vi "Configure PID Differential Time.vi"(8 "error in (no error)":errorcluster, 10 "differential time, s":dbl, 11 "HECR in":refnum<class "PL SMC HECR.lvclass">) -> (0 "error out":errorcluster, 3 "HECR out":refnum<class "PL SMC HECR.lvclass">)   [LabVIEW 2015, in "PL SMC HECR.lvclass"]
doc: "Configures PID differential time."
uses:
  PL SMC HECR.lvclass
  <vilib>/plasmapper/PL Modbus Client/PL Modbus Client.lvclass
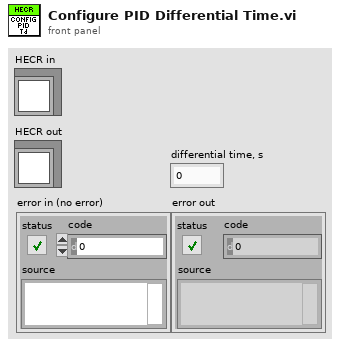
[diagram p1: front panel]
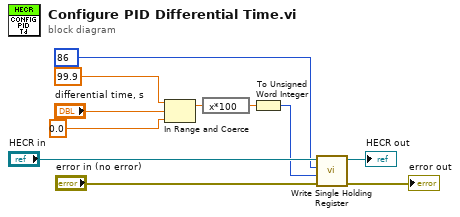
[diagram p0: block diagram]
diagram:
  n1 = In Range and Coerce(upper limit=99.9 ("Ttarget, °C"), x="differential time, s", lower limit=0.0 ("Ttarget, °C")) -> (coerced(x)=w2:dbl)  [unwired: 1 out]
  n2 = expression code="x*100"(w2) -> (w1:dbl)
  n3 = To Unsigned Word Integer(number=w1) -> (unsigned 16bit integer=w3:u16)
  n4 = call <vilib>:"Write Single Holding Register.vi"("error in (no error)"="error in (no error)", "value"=w3, "address"=u16 86, "MODBUS in"="HECR in") -> ("error out"=→"error out":errorcluster, "MODBUS out"=→"HECR out":refnum<class "PL SMC HECR.lvclass">)  [unwired: 6 in]
